vi "Exercise 5-2.vi"() -> ()   [LabVIEW 2014]
panel:
  out "Small Cluster":cluster{"Boolean 1":bool, "Slide Value":dbl}
  out "Modified Cluster":T1 {"Slide" scale=0.0..10.0}
  in  "Cluster":T1 {"Slide" scale=0.0..10.0}
  out "Boolean 2":bool
  out "Numeric":dbl
  in  "?":bool
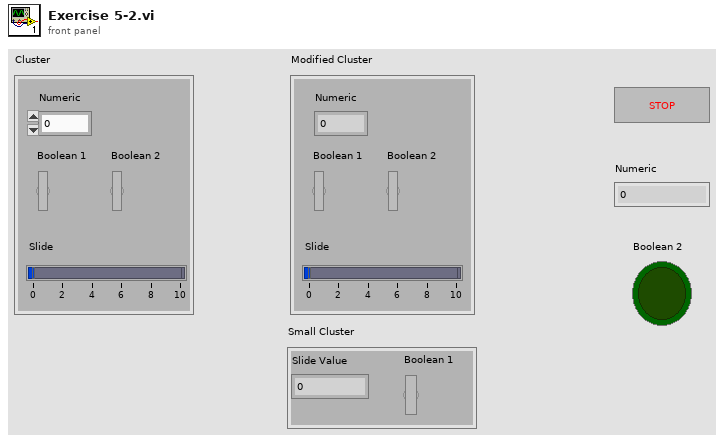
[diagram p1: front panel]
types:
  T1 = cluster{"Numeric":dbl, "Boolean 1":bool, "Boolean 2":bool, "Slide":dbl}
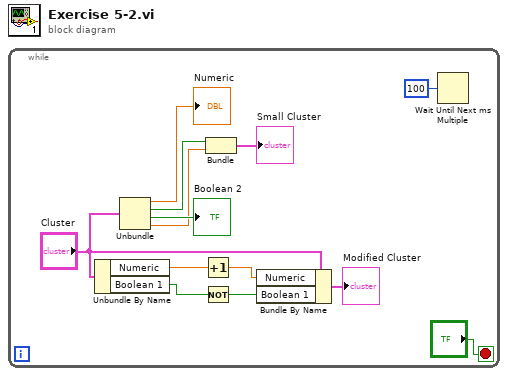
[diagram p0: block diagram]
diagram:
  n1 = while {
    stop <- "?" stop-if-true
    n2 = Unbundle By Name("Cluster") -> ("Numeric"=w5:dbl, "Boolean 1"=w3:bool)
    n3 = Unbundle("Cluster") -> ("Numeric"=→"Numeric":dbl, "Boolean 1"=w10:bool, "Boolean 2"=→"Boolean 2":bool, "Slide"=w8:dbl)
    n4 = Increment(x=w5) -> (x+1=w4:dbl)
    n5 = Not(x=w3) -> (.not. x?=w2:bool)
    n6 = Bundle("Boolean 1"=w10, "Slide"=w8) -> (→"Small Cluster":cluster{"Boolean 1":bool, "Slide":dbl})  [unwired: 1 in]
    n7 = Bundle By Name(cluster="Cluster", "Numeric"=w4, "Boolean 1"=w2) -> (→"Modified Cluster":T1)
    n8 = Wait Until Next ms Multiple(millisecond multiple=u32 100) -> ()  [unwired: 1 out]
  }
